vi "config okay.vi"(10 "error in (no error)":errorcluster) -> (2 "error out":errorcluster, 3 "config okay":bool)   [LabVIEW 2012]
uses:
  ReadWrite.ctl
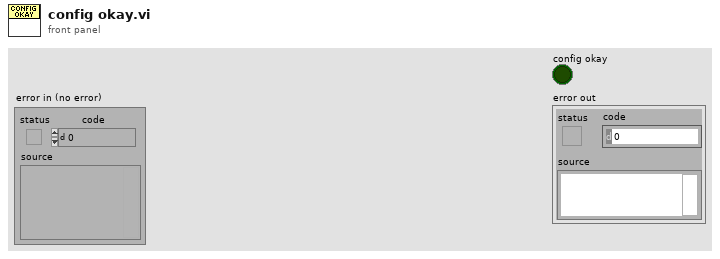
[diagram p1: front panel]
types:
  T1 = typedef "ReadWrite.ctl" = enum16{"Read", "Write"}
  T2 = typedef "SVN.ctl" = cluster{"Mathcad Code Repository":string, "Username":string, "Password":string, "Method file names (w extension)":string}
  T3 = typedef "Paths.ctl" = cluster{"Mathcad Methods":path, "Requested Designs":path, "Completed Designs":path, "Mathcad Code":path, "Collabnet SVN":path, "Mathcad Methods ok":bool, "Requested Designs ok":bool, "Completed Designs ok":bool, "Mathcad Code ok":bool, "Collabnet SVN":bool}
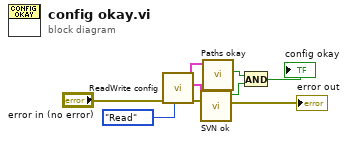
[diagram p0: block diagram]
diagram:
  n1 = call "ReadWrite config.vi"("Config"=ReadWrite."Read", "error in (no error)"="error in (no error)") -> ("error out"=w4:errorcluster, "SVN"=w8:T2, "Paths"=w7:T3)  [unwired: 6 in, 1 out]
  n2 = call "SVN ok.vi"("error in"=w4, "SVN in"=w8) -> ("error out"=→"error out":errorcluster, "SVN ok"=w5:bool)  [unwired: 8 in]
  n3 = call "Paths okay.vi"("Paths"=w7) -> ("passed"=w6:bool)  [unwired: 9 in, 1 out]
  n4 = And(x=w6, y=w5) -> (x .and. y?=→"config okay":bool)
